vi "zad3.vi"() -> ()   [LabVIEW 2017]
panel:
  out "Licznik":i16
  in  "?":bool
  in  "String":string
  in  "Numeric Control":i64
  in  "Blank Button":bool
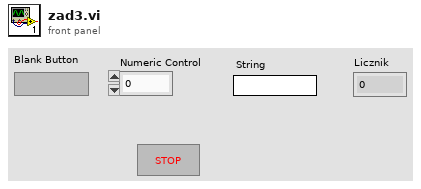
[diagram p1: front panel]
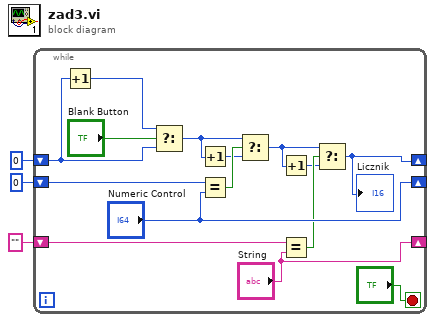
[diagram p0: block diagram]
diagram:
  n1 = while {
    shift-right: [w7] -> _
    shift-left: 0 -> [w13]
    shift-right: ["Numeric Control"] -> _
    shift-left: 0 -> [w16]
    shift-right: ["String"] -> _
    shift-left: "" -> [w9]
    stop <- "?" stop-if-true
    n2 = Increment(x=w13) -> (x+1=w12:i32)
    n3 = Select(t=w12, s="Blank Button", f=w13) -> (s? t:f=w11:i32)
    n4 = Increment(x=w11) -> (x+1=w10:i32)
    n5 = Equal?(x=w16, y="Numeric Control") -> (x = y?=w15:bool)
    n6 = Select(t=w11, s=w15, f=w10) -> (s? t:f=w5:i32)
    n7 = Increment(x=w5) -> (x+1=w4:i32)
    n8 = Equal?(x=w9, y="String") -> (x = y?=w8:bool)
    n9 = Select(t=w5, s=w8, f=w4) -> (s? t:f=w7:i32)
    "Licznik" <- w7
  }
